vi "Tracepoint_TagError.vi"(8 "error in (no error)":errorcluster, 9 "log string":string, 10 "Error":bool, 11 "Qbus":refnum<class "Qbus.lvclass">) -> (0 "error out":errorcluster)   [LabVIEW 2017, in "OPCUAClient.lvlib"]
uses:
  <vilib>/addons/InsightCM/Devices/Shared/Common/OPCUAClient/OPCUAClient.lvlib
  <vilib>/addons/Qbus/Qbus.lvclass
  <vilib>/addons/TraceLogger/TraceLogger.lvlib
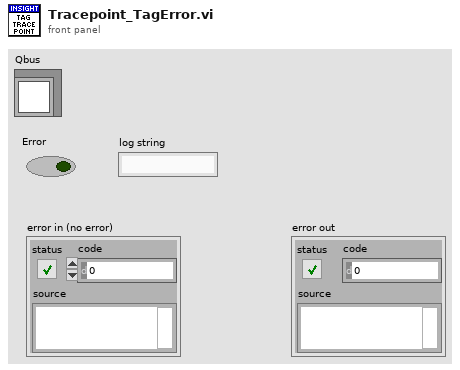
[diagram p1: front panel]
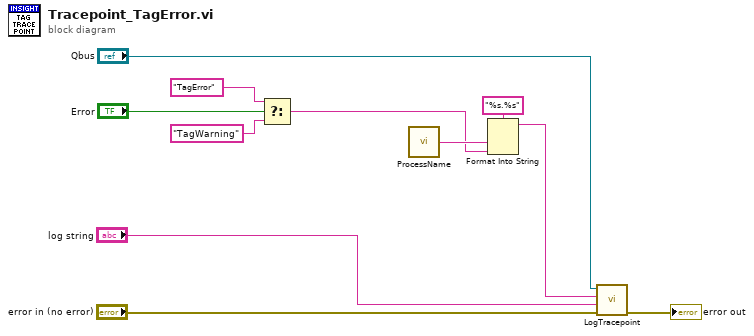
[diagram p0: block diagram]
diagram:
  n1 = Select(t="TagError" ("tracepoint"), s="Error", f="TagWarning" ("tracepoint")) -> (s? t:f=w4:string)
  n2 = call <vilib>:"ProcessName.vi"() -> ("process name"=w8:string)  [unwired: 5 in]
  n3 = Format Into String(format string="%s.%s", w8, w4) -> (resulting string=w3:string)  [unwired: 2 in, 1 out]
  n4 = call <vilib>:"LogTracepoint.vi"("error in (no error)"="error in (no error)", "log string"="log string", "tracepoint"=w3, "qbus in"="Qbus") -> ("error out"=→"error out":errorcluster)  [unwired: 6 in, 1 out]
